vi "Global-trigger.vi"() -> ()   [LabVIEW 2020]
panel:
  in  "global trigger":bool
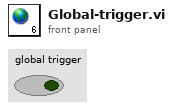
[diagram p1: front panel]
diagram:
